vi "1.3nad.vi"() -> ()   [LabVIEW 2020]
uses:
  <vilib>/numeric/Random Number (Range) I64.vi
  <vilib>/numeric/sub_Random U32.vi
panel:
  out "Waveform Chart":i32(graph)
  in  "stop":bool
  out "Numeric":i64
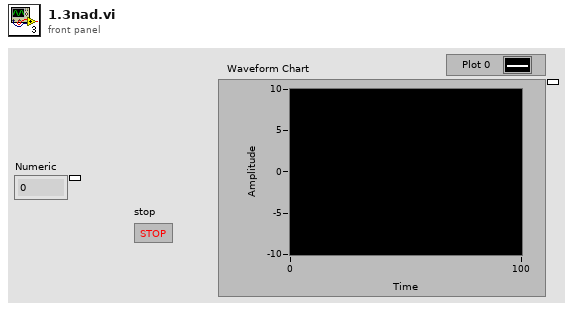
[diagram p1: front panel]
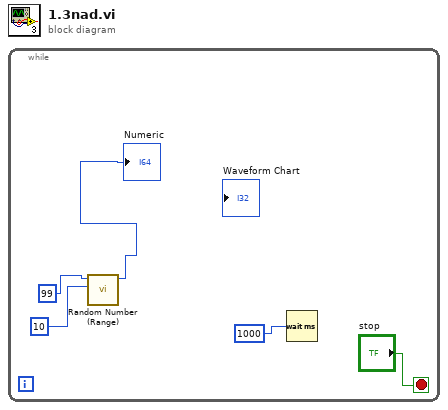
[diagram p0: block diagram]
diagram:
  n1 = while {
    stop <- "stop" stop-if-true
    n2 = call-poly <vilib>:"Random Number (Range).vi"("lower bound (-100)"=10, "upper bound (100)"=99) -> ("number"=→"Numeric":i64)  [unwired: 9 in]
    n3 = Wait (ms)(milliseconds to wait=1000) -> ()  [unwired: 1 out]
  }
